vi "Read Value.vi"(8 "error in (no error)":errorcluster, 11 "ConvertTo_DBL in":refnum<class "ConvertTo_SGL.lvclass">) -> (0 "error out":errorcluster, 2 "Abs_Numeric.lvclass":refnum<class "Abs_Numeric.lvclass">, 3 "ConvertTo_DBL out":refnum<class "ConvertTo_SGL.lvclass">)   [LabVIEW 2021, in "ConvertTo_SGL.lvclass"]
uses:
  ConvertTo_SGL.lvclass
  Abs_Types/Numeric/Abs_Numeric.lvclass
  ConvertTo_SGL.lvclass/ConvertTo_SGL.ctl
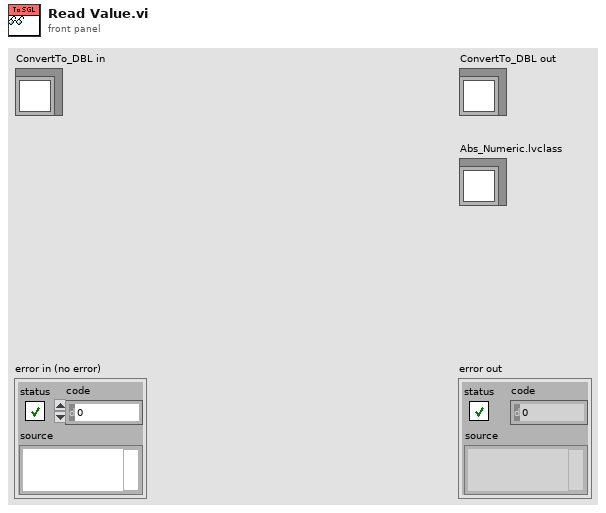
[diagram p1: front panel]
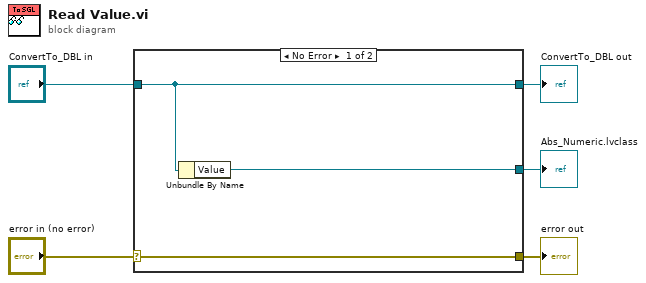
[diagram p0: block diagram]
diagram:
  n1 = case shown="No Error" "error in (no error)" {
    selector: "error in (no error)" -> [w8 w9]
    tunnel: [w8 w9] -> w4
    tunnel: [w7 w10] -> w2
    tunnel: "ConvertTo_DBL in" -> [w7 w10]
    tunnel: [w6 _] -> w1
    frame No Error {
      n2 = Unbundle By Name(w7) -> ("Value"=w6:refnum<class "Abs_Numeric.lvclass">)
    }
    frame Error {
    }
  }
  "error out" <- w4
  "ConvertTo_DBL out" <- w2
  "Abs_Numeric.lvclass" <- w1
